vi "HumidityNewton.vi"(8 "error in (no error)":errorcluster) -> (0 "error out":errorcluster, 2 "Cashew Humidity":dbl(knob) scale=0.0..120.0)   [LabVIEW 2018]
uses:
  <vilib>/express/express arith-compare/Formula/XNode/ExpressFormulaBlockNode.xnode
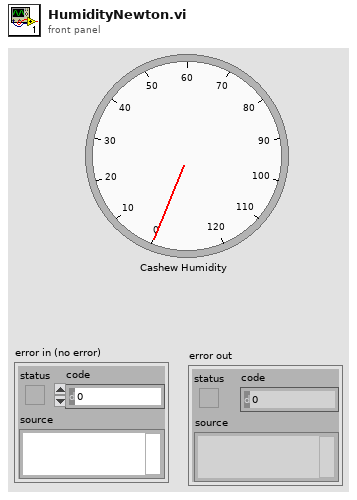
[diagram p1: front panel]
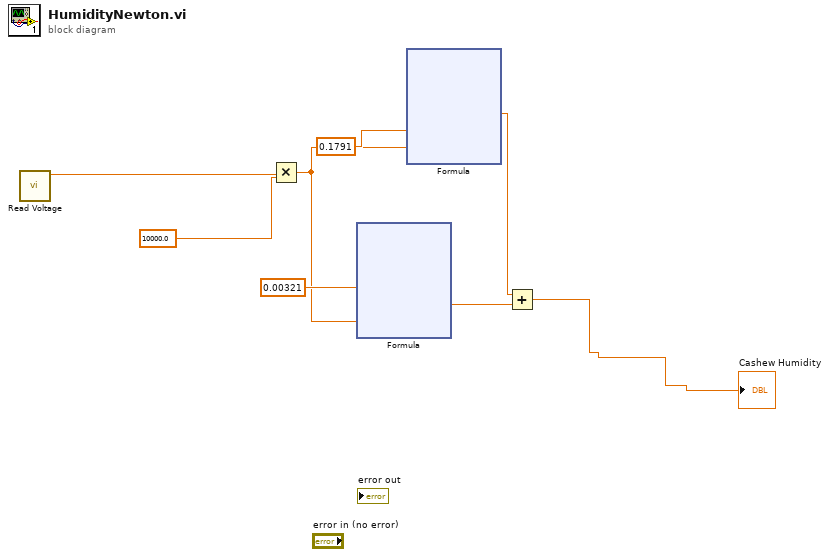
[diagram p0: block diagram]
diagram:
  n1 = call "Read Voltage.vi"() -> ("voltage"=w8:dbl)  [unwired: 1 in, 6 out]
  n2 = Multiply(x=w8, y=10000.0) -> (x*y=w4:dbl)
  n3 = xnode "Formula"("b"=0.00321, "t"=w4) -> ("Result"=w2:dbl)  [unwired: 1 in, 1 out]
  n4 = xnode "Formula"("K"=0.1791, "t"=w4) -> ("Result"=w3:dbl)  [unwired: 1 in, 1 out]
  n5 = Add(x=w3, y=w2) -> (x+y=→"Cashew Humidity":dbl)
